vi "SaveTestAs.vi"(8 "error in (no error)":errorcluster, 10 "Value":string, 11 "TreeControl in":refnum<vi>) -> (0 "error out":errorcluster, 1 "Cancelled?":bool)   [LabVIEW 2018]
uses:
  Tree/Controls/Plugins Tree Item Type.ctl
panel:
  in  "Cancel Button":bool
  in  "OK Button":bool
  in  "Test Name":string
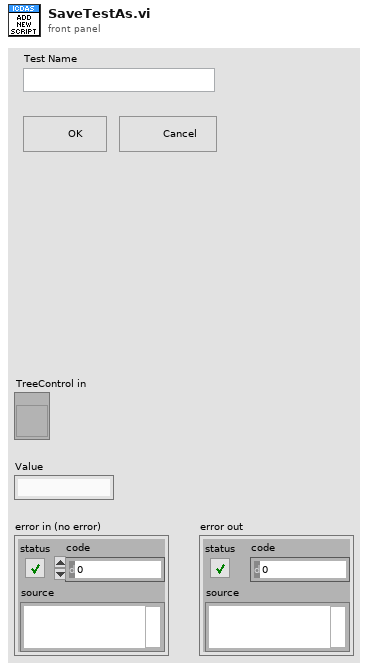
[diagram p1: front panel]
types:
  T1 = typedef "Plugins Tree Item Type.ctl" = enum16{"Plugin", "Instrument", "INI File", "INI Script"}
  T2 = typedef "Plugin Tree Tag.ctl" = cluster{"ItemType":T1, "Name":string, "Path":path, "Script":string[]}
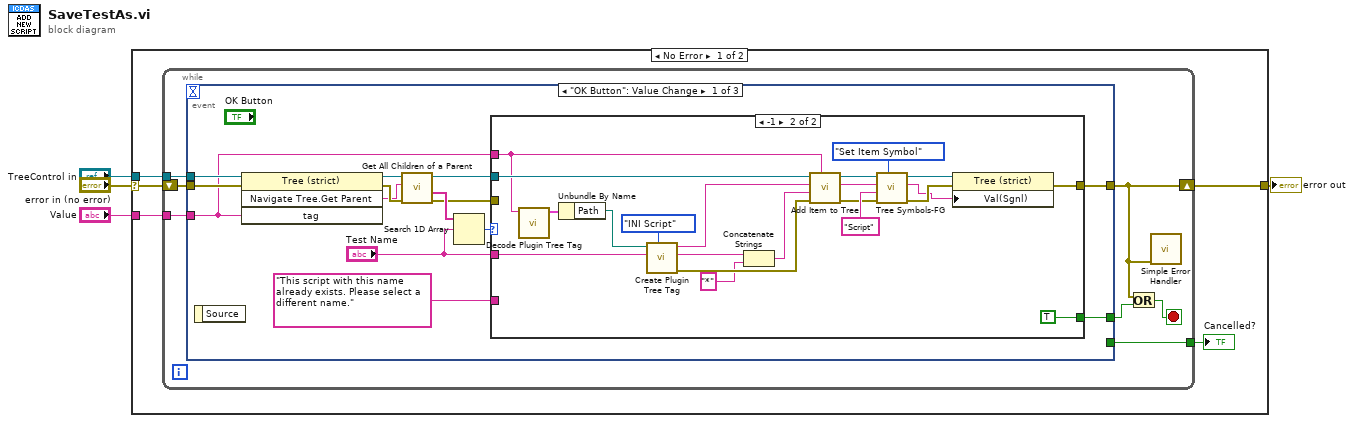
[diagram p0: block diagram]
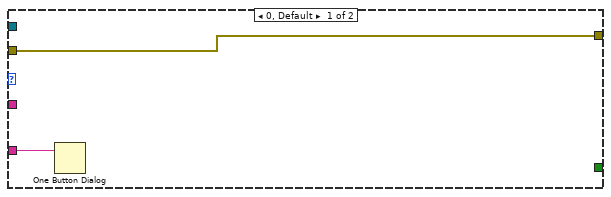
[diagram p2: hidden frame]
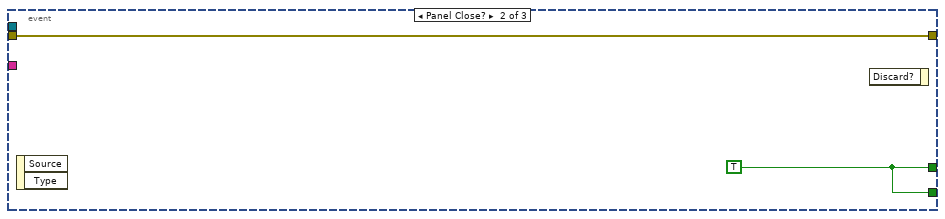
[diagram p3: hidden frame]
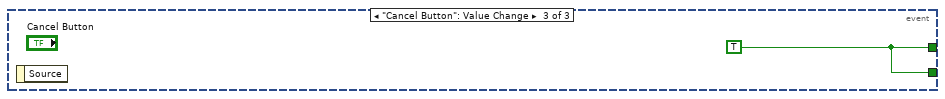
[diagram p4: hidden frame]
diagram:
  n1 = case shown="No Error" "error in (no error)" {
    selector: "error in (no error)" -> [w6 w57]
    tunnel: [w9 w57] -> w4
    tunnel: "Value" -> [w8 _]
    tunnel: "TreeControl in" -> [w7 _]
    frame No Error {
      n2 = while {
        tunnel: w8 -> [w16]
        tunnel: w7 -> [w15]
        shift-right: [w11] -> w9
        shift-left: w6 -> [w14]
        tunnel: [w10] -> w5
        stop <- w12 stop-if-true
        n3 = event shown="[0] \"OK Button\": Value Change" {
          selector: _ -> [_ _ _]
          dyn-events: _ -> [_ _ _]
          timeout: _ -> [_ _ _]
          tunnel: [w20 w55 _] -> w11
          tunnel: w16 -> [w17 _ _]
          tunnel: w15 -> [w30 _ _]
          tunnel: w14 -> [w29 w55 _]
          tunnel: [w22 w54 w56] -> w13
          tunnel: [_ w54 w56] -> w10
          event "OK Button": Value Change {
            n4 = event-data() -> ()  [unwired: 1 in, 1 out]
            n5 = invoke class="Tree (strict)" method="Navigate Tree.Get Parent"(reference=w30, error in=w29, "tag"=w17) -> (reference out=w28:refnum<vi>, error out=w27:errorcluster, "Navigate Tree:Get Parent"=w18:string)  [unwired: 1 in, 1 out]
            n6 = call "Get All Children of a Parent.vi"("Error In"=w27, "Parent tag"=w18, "Tree ref"=w28) -> ("Error out"=w19:errorcluster, "All Children"=w26:string[], "Tree ref out"=w25:refnum<vi>)  [unwired: 5 in, 1 out]
            n7 = Search 1D Array(1D array=w26, element="Test Name") -> (index of element=w24:i32)  [unwired: 1 in]
            n8 = case shown="-1" w24 {
              tunnel: w17 -> [_ w40]
              tunnel: w25 -> [_ w44]
              tunnel: "This script with this name already exists. Please select a different name." ("Script Name") -> [w32 _]
              tunnel: [_ TRUE] -> w22
              tunnel: "Test Name" -> [_ w33]
              tunnel: [w31 w38] -> w20
              tunnel: w19 -> [w31 _]
              frame 0, Default {
                n9 = One Button Dialog(message=w32) -> ()  [unwired: 1 in, 1 out]
              }
              frame -1 {
                n10 = call "Decode Plugin Tree Tag.vi"("Tag"=w40) -> ("Plugin Tree Tag"=w43:T2)  [unwired: 9 in, 1 out]
                n11 = Unbundle By Name(w43) -> ("Path"=w42:path)
                n12 = call "Create Plugin Tree Tag.vi"("ItemType"=Plugins_Tree_Item_Type."INI Script", "Name"=w33, "VISA Resource"=w42) -> ("error out"=w52:errorcluster, "Name out"=w34:string, "Tag"=w46:string)  [unwired: 6 in]
                n13 = Concatenate Strings(w34, "*" ("string")) -> (w35:string)
                n14 = call "Add Item to Tree.vi"("Parent Tag"=w40, "error in (no error)"=w52, "Item Name"=w35, "Item Tag"=w46, "Tree Ref"=w44) -> ("error out"=w47:errorcluster, "Item Tag out"=w49:string, "reference out"=w48:refnum<vi>)  [unwired: 3 in, 1 out]
                n15 = call "Tree Symbols-FG.vi"("Actions"=enum16{"Init Symbols", "Set Item Symbol"}."Set Item Symbol", "error in (no error)"=w47, "Symbol Name"="Script", "Item Tag"=w49, "Tree Ref"=w48) -> ("error out"=w41:errorcluster, "Item Tag out"=w36:string, "Tree Ref out"=w37:refnum<vi>)  [unwired: 4 in]
                n16 = property class="Tree (strict)"(reference=w37, error in=w41, "Val(Sgnl)"=w36) -> (error out=w38:errorcluster)  [unwired: 1 out]
              }
            }
          }
          event Panel Close? {
            w54 = TRUE
            n17 = event-data() -> ()  [unwired: 1 in, 2 out]
            n18 = event-data() -> ()  [unwired: 2 in, 1 out]
          }
          event "Cancel Button": Value Change {
            w56 = TRUE
            n19 = event-data() -> ()  [unwired: 1 in, 1 out]
          }
        }
        n20 = Or(x=w11, y=w13) -> (x .or. y?=w12:bool)
        n21 = call <vilib>:"Simple Error Handler.vi"("error in (no error)"=w11) -> ()  [unwired: 4 in, 5 out]
      }
      "Cancelled?" <- w5
    }
    frame Error {
    }
  }
  "error out" <- w4
